vi "class_data.vi"() -> ()   [LabVIEW 2010, in "FPGAWrapperRK110909Throughput.lvclass"]
uses:
  FPGAWrapperRK110909Throughput.lvclass
  FPGA_reference.ctl
panel:
  out "FPGA Interface":T1
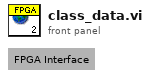
[diagram p1: front panel]
types:
  T1 = typedef "FPGAWrapperRK110909Throughput.lvclass/FPGA_reference.ctl" = refnum<k20>
diagram:
